vi "CSConnectGUI.panel.vi"() -> ()   [LabVIEW 2014, in "CSConnectGUI.lvlib"]
doc: "GUI for the CSConnector class (and its children)\n\nauthor: Dennis Neidherr, GSI\nlicense: GPL"
uses:
  CSConnectGUI.lvlib
  CSlibraries-extern/DimLVEvent/DimIndicators/DimIndicators.numericType.ctl
  CSlibraries-extern/DimLVEvent/DimIndicators/DimIndicators.anyType.ctl
  CSlibraries-extern/DimLVEvent/DimIndicators/DimIndicators.numericArrayType.ctl
  CSlibraries/UtilityLib/UtilityLib.valueStatus.ctl
  CSlibraries/UtilityLib/UtilityLib.helpType.ctl
  CSCore/CSSystem/CoreLib/CoreLib.short 2 byte array.vi
  CSCore/CSSystem/CoreLib/CoreLib.double 2 byte array.vi
  CSCore/CSSystem/CoreLib/CoreLib.lvlib
  CSlibraries/UtilityLib/UtilityLib.lvlib
  CSlibraries-extern/DimLVEvent/DimIndicators/DimIndicators.lvlib
  CSCore/CSApplicationBaseClasses/DeviceBase/DeviceBase.lvlib
  CSCore/GUIs/GOGUserGUIs/DeviceBaseGUI/DeviceBaseGUI.lvlib
  CSCore/CSObj/CSObj.lvlib
  CSlibraries-extern/DimLVEvent/LVDimInterface/LVDimInterface.lvlib
panel:
  in  "actStatus15":T1
  in  "actStatus14":T1
  in  "actStatus13":T1
  in  "actStatus12":T1
  in  "actStatus11":T1
  in  "actStatus10":T1
  in  "actStatus9":T1
  in  "actStatus8":T1
  in  "actStatus7":T1
  in  "actStatus6":T1
  in  "actStatus5":T1
  in  "actStatus4":T1
  in  "actStatus3":T1
  in  "actStatus2":T1
  in  "actStatus1":T1
  in  "actStatus0":T1
  out "channelIndex":u16
  in  "nomOutVoltages15":T1
  in  "nomOutVoltages14":T1
  in  "nomOutVoltages13":T1
  in  "nomOutVoltages12":T1
  in  "nomOutVoltages11":T1
  in  "nomOutVoltages10":T1
  in  "nomOutVoltages9":T1
  in  "nomOutVoltages8":T1
  in  "nomOutVoltages7":T1
  in  "nomOutVoltages6":T1
  in  "nomOutVoltages5":T1
  in  "nomOutVoltages4":T1
  in  "nomOutVoltages3":T1
  in  "nomOutVoltages2":T1
  in  "nomOutVoltages1":T1
  in  "nomOutVoltages0":T1
  in  "actOutVoltages15":T1
  in  "actOutVoltages14":T1
  in  "actOutVoltages13":T1
  in  "actOutVoltages12":T1
  in  "actOutVoltages11":T1
  in  "actOutVoltages10":T1
  in  "actOutVoltages9":T1
  in  "actOutVoltages8":T1
  in  "actOutVoltages7":T1
  in  "actOutVoltages6":T1
  in  "actOutVoltages5":T1
  in  "actOutVoltages4":T1
  in  "actOutVoltages3":T1
  in  "actOutVoltages2":T1
  in  "actOutVoltages1":T1
  in  "actOutVoltages0":T1
  in  "function":u16(ring)
  in  "EmergencyOff":bool
  in  "Set":bool
  in  "inc":dbl
  in  "setValue":dbl format="%^#_9e"
  out "ErrorString":string
  out "Busy":bool
  in  "logicalNames":T2 caption="dic_service_anyType"
  in  "nofChannels":T3 caption="dic_service_numeric"
  in  "nomVoltage":T1 caption="dic_service_numericArray"
  out "deviceIDString":string
  in  "tab":enum32{"standard"}(tab)
  in  "standardDisplay":i32[](listbox)
  in  "minus":bool
  in  "plus":bool
  out "loop counter":i32
  out "error out":errorcluster
  in  "error in (no error)":errorcluster
  in  "object ref":refnum<vi>
  in  "state":T3 caption="dic_service_numeric"
  in  "deviceID":T2 caption="dic_service_anyType"
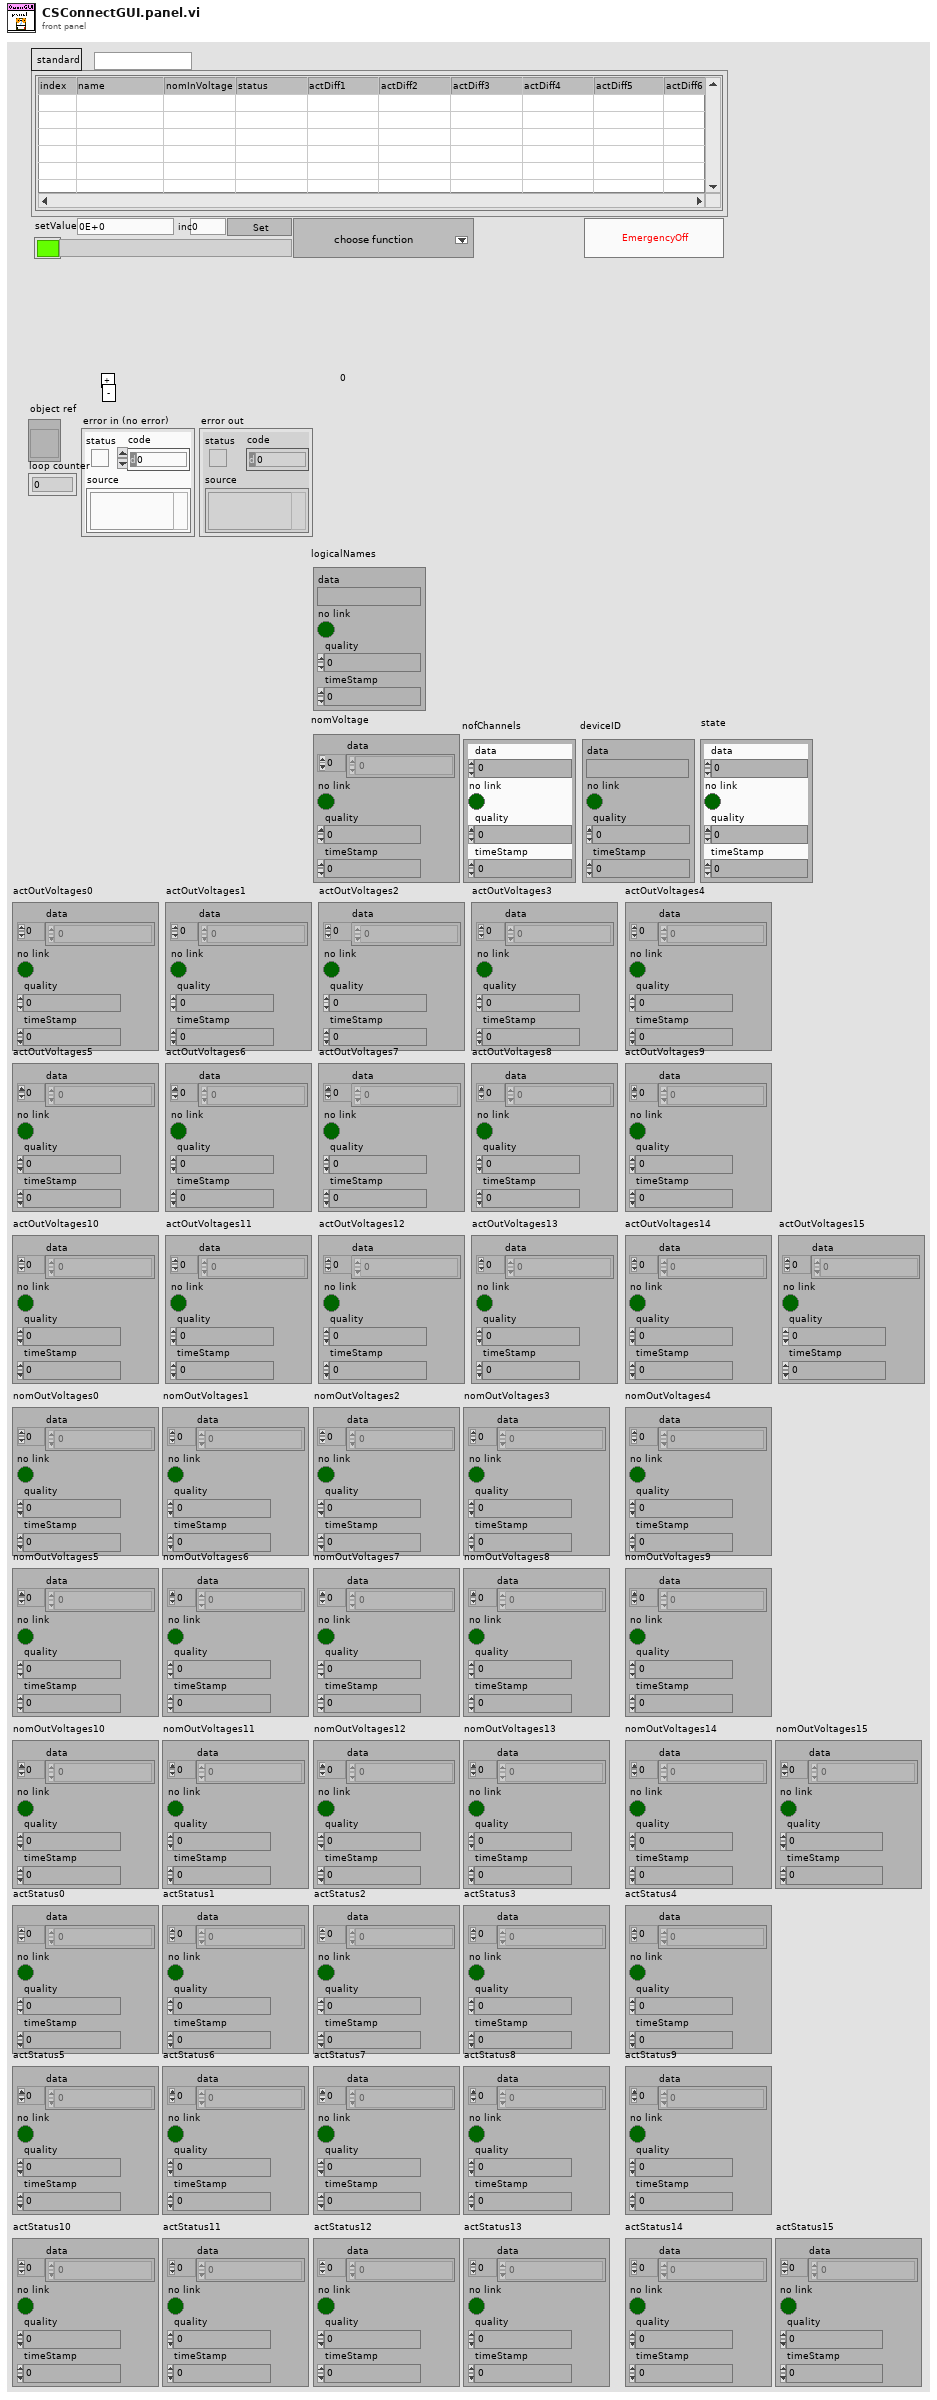
[diagram p1: front panel]
types:
  T1 = typedef "DimIndicators.lvlib/DimIndicators.numericArrayType.ctl" = cluster{"data":dbl[], "no link":bool, "quality":i32, "timeStamp":dbl}
  T2 = typedef "DimIndicators.lvlib/DimIndicators.anyType.ctl" = cluster{"data":string, "no link":bool, "quality":i32, "timeStamp":dbl}
  T3 = typedef "DimIndicators.lvlib/DimIndicators.numericType.ctl" = cluster{"data":dbl, "no link":bool, "quality":i32, "timeStamp":dbl}
  T4 = typedef "UtilityLib.lvlib/UtilityLib.valueStatus.ctl" = enum16{"no info available", "stand by/off", "on", "warning", "alarm/malfunction", "not implemented", "user action required", "important information", "system default", "control default", "indicator default", "button default"}
  T5 = cluster{"ObjectIndex":i32, "OutChannelIndex":i32}
  T6 = typedef "UtilityLib.lvlib/UtilityLib.helpType.ctl" = enum16{"unknown", "menu", "description", "about", "special0", "special1", "special2"}
  T7 = cluster{"ObjectName":string, "Indizes":cluster{"Index":i32, "Position in Matrix":i32}[]}[]
  T8 = typedef "DeviceBaseGUI.lvlib/DeviceBaseGUI.i attribute.ctl" = cluster{"GOGFrontPanel.i attribute":T9}
  T9 = typedef "GOGFrontPanel.lvlib/GOGFrontPanel.i attribute.ctl" = cluster{"GOGObject":string, "Object":string, "Method":string, "Descriptor":T10, "Input Descriptor":string, "Output Descriptor":string, "inputNames":string[], "outputNames":string[], "Values":cluster{"descriptor":string, "value":string}[]}
  T10 = typedef "BaseProcess.lvlib/BaseProcess.descriptor string definition.ctl" = string
  T11 = cluster{"ObjectName":string, "Indizes":cluster{"Index":i32, "Position in Matrix":i32}[]}
  T12 = typedef "LVRectTypeDef.ctl" = cluster{"Left":i16, "Top":i16, "Right":i16, "Bottom":i16}
  T13 = typedef "CoreDefs.rawDataType.ctl" = i8[]
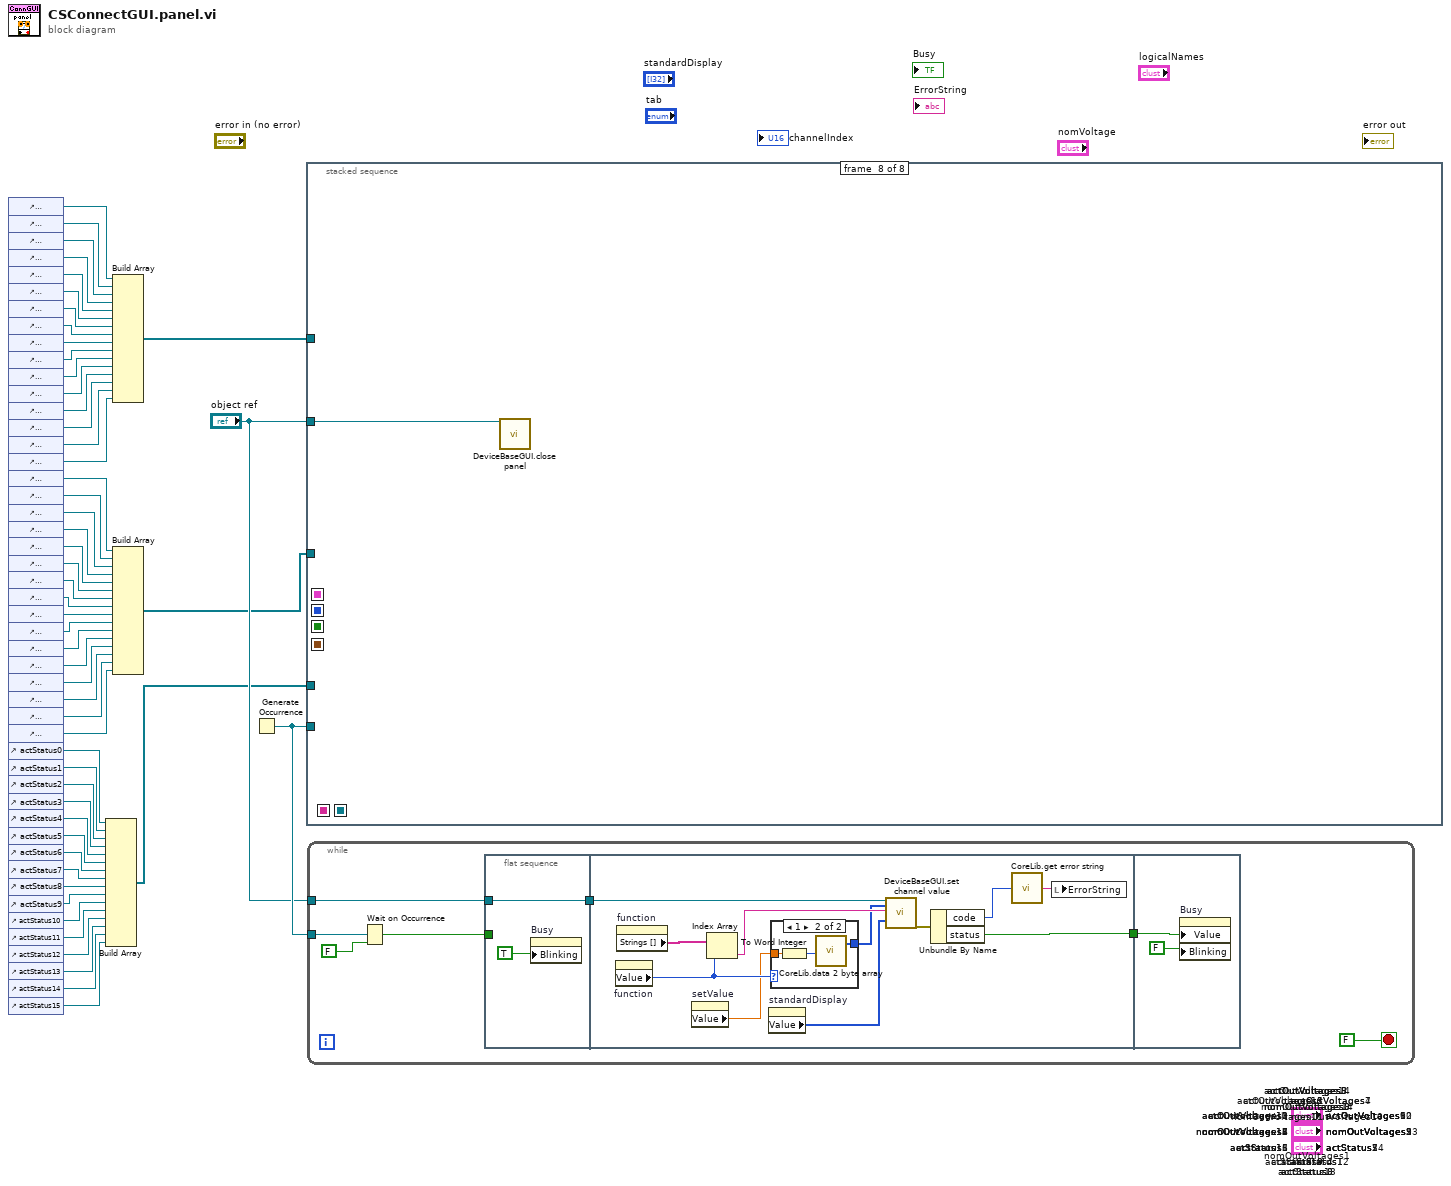
[diagram p0: block diagram]
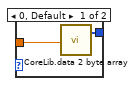
[diagram p2: hidden frame]
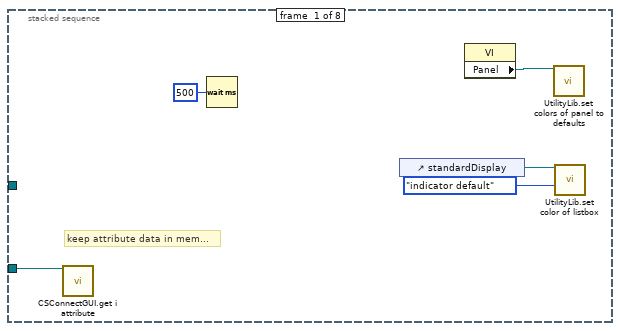
[diagram p3: hidden frame]
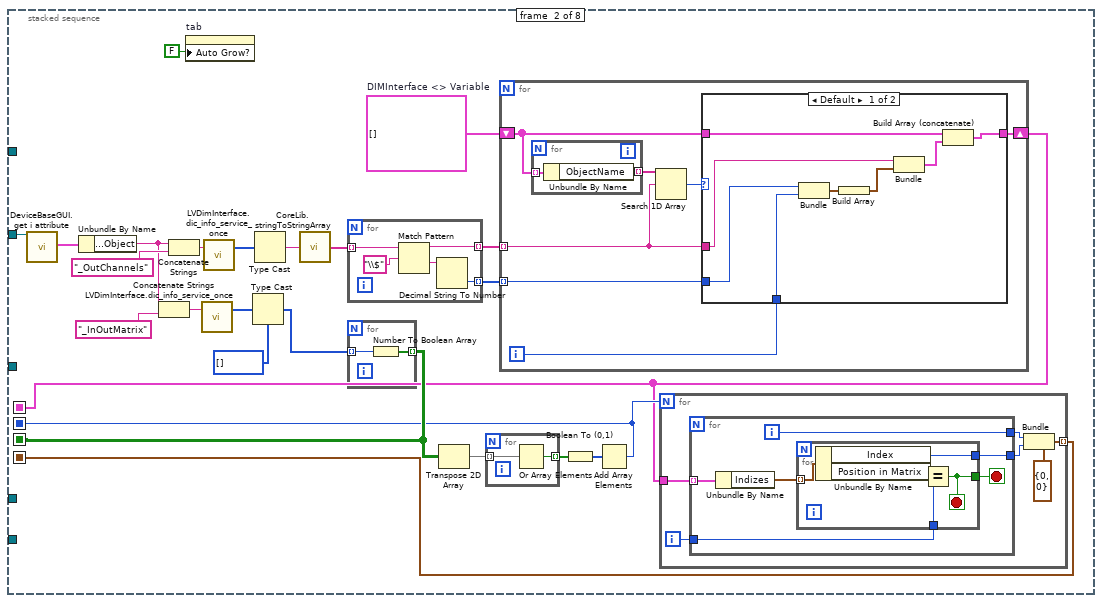
[diagram p4: hidden frame]
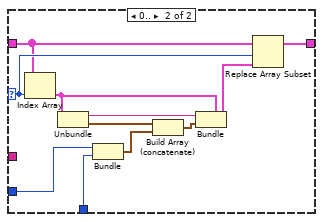
[diagram p5: hidden frame]
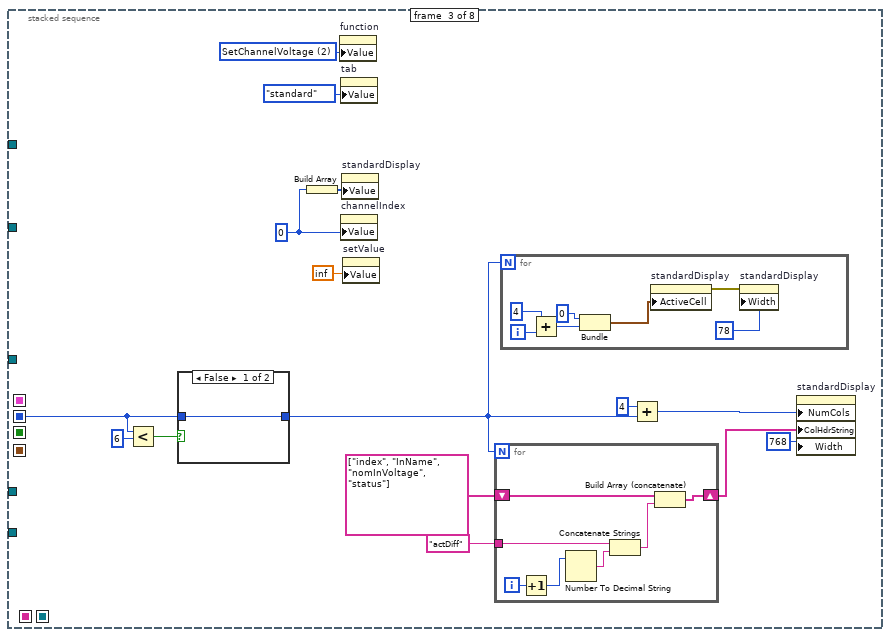
[diagram p6: hidden frame]
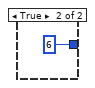
[diagram p7: hidden frame]
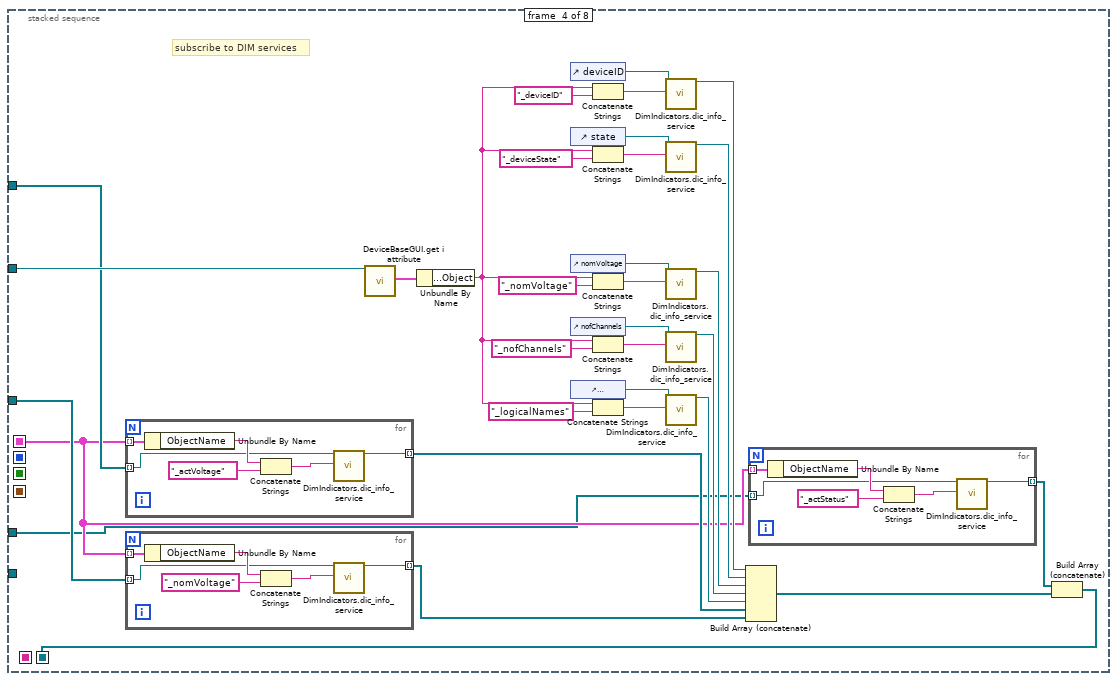
[diagram p8: hidden frame]
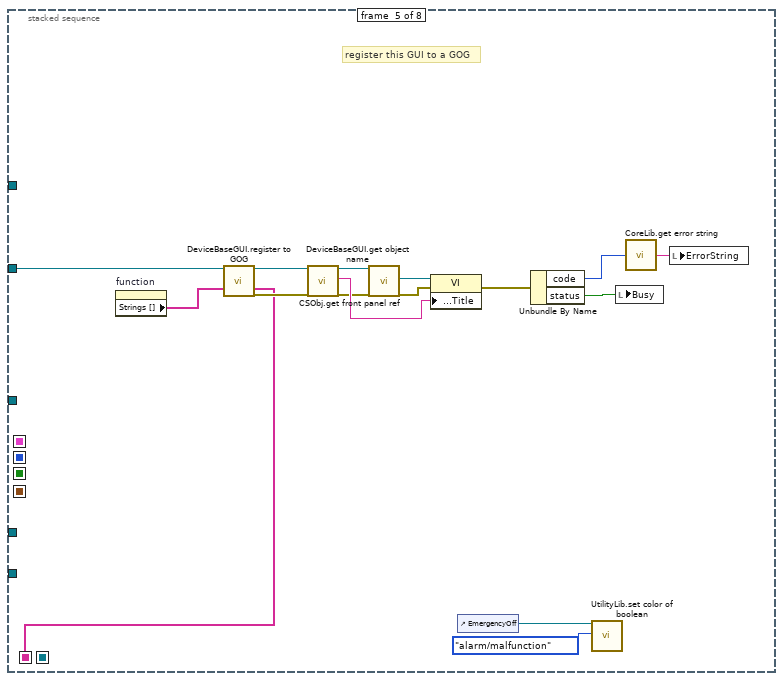
[diagram p9: hidden frame]
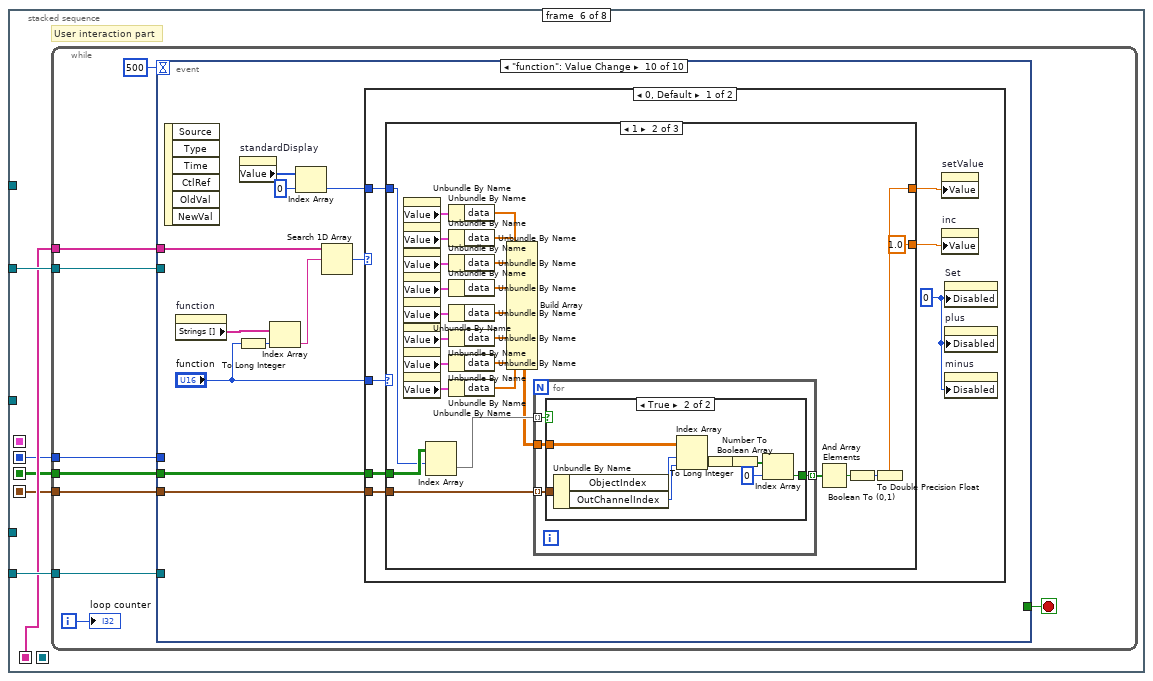
[diagram p10: hidden frame]
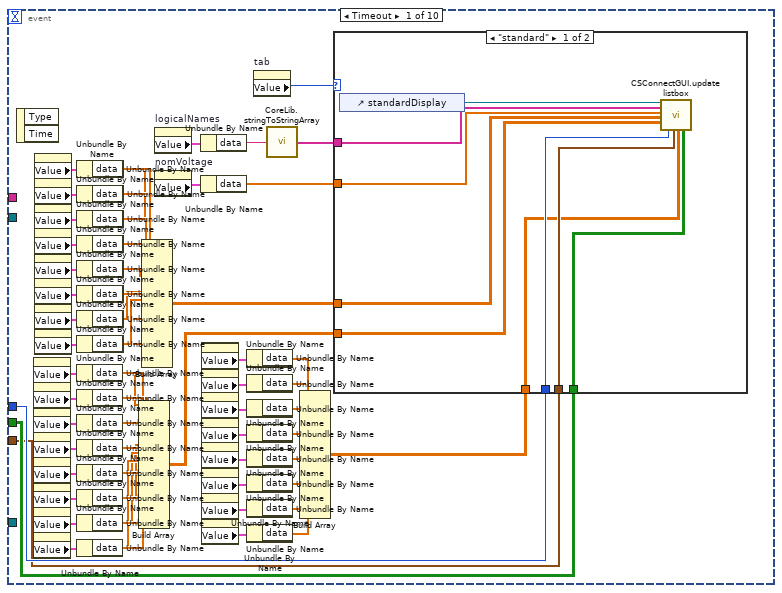
[diagram p11: hidden frame]
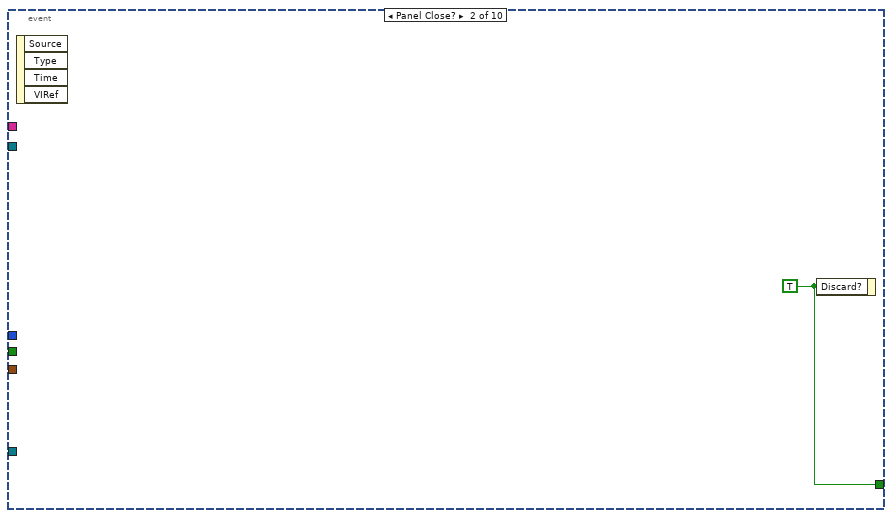
[diagram p13: hidden frame]
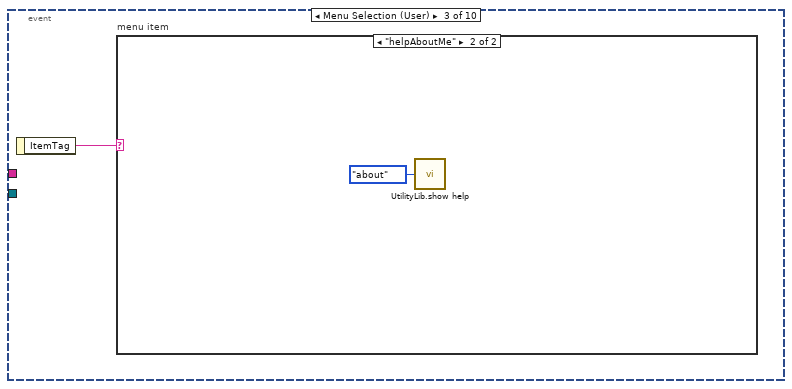
[diagram p14: hidden frame]
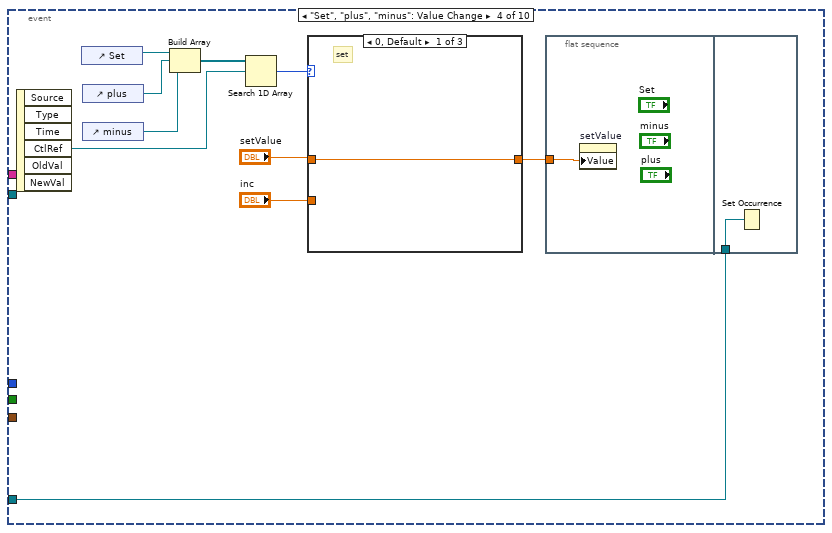
[diagram p16: hidden frame]
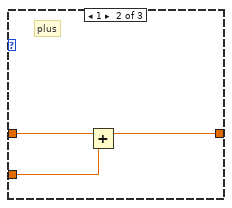
[diagram p17: hidden frame]
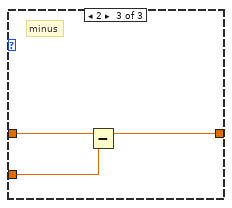
[diagram p18: hidden frame]
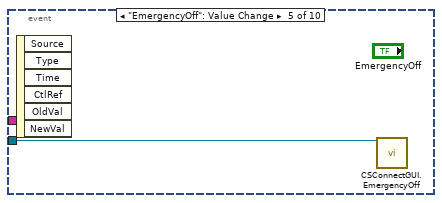
[diagram p19: hidden frame]
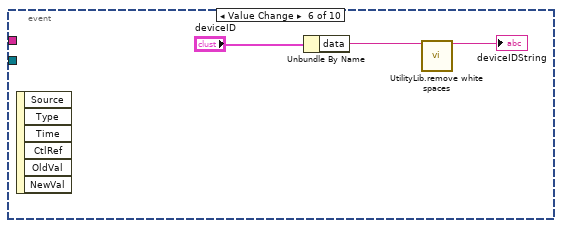
[diagram p20: hidden frame]
diagram:
  n1 = control-ref of="actOutVoltages0"() -> (w51:refnum<vi>)
  n2 = control-ref of="actOutVoltages1"() -> (w50:refnum<vi>)
  n3 = control-ref of="actOutVoltages2"() -> (w49:refnum<vi>)
  n4 = control-ref of="actOutVoltages3"() -> (w48:refnum<vi>)
  n5 = control-ref of="actOutVoltages4"() -> (w47:refnum<vi>)
  n6 = control-ref of="actOutVoltages5"() -> (w46:refnum<vi>)
  n7 = control-ref of="actOutVoltages6"() -> (w45:refnum<vi>)
  n8 = control-ref of="actOutVoltages7"() -> (w44:refnum<vi>)
  n9 = control-ref of="actOutVoltages8"() -> (w43:refnum<vi>)
  n10 = control-ref of="actOutVoltages9"() -> (w42:refnum<vi>)
  n11 = control-ref of="actOutVoltages10"() -> (w41:refnum<vi>)
  n12 = control-ref of="actOutVoltages11"() -> (w36:refnum<vi>)
  n13 = control-ref of="actOutVoltages12"() -> (w37:refnum<vi>)
  n14 = control-ref of="actOutVoltages13"() -> (w38:refnum<vi>)
  n15 = control-ref of="actOutVoltages14"() -> (w39:refnum<vi>)
  n16 = control-ref of="actOutVoltages15"() -> (w40:refnum<vi>)
  n17 = control-ref of="nomOutVoltages0"() -> (w34:refnum<vi>)
  n18 = control-ref of="nomOutVoltages1"() -> (w33:refnum<vi>)
  n19 = control-ref of="nomOutVoltages2"() -> (w32:refnum<vi>)
  n20 = control-ref of="nomOutVoltages3"() -> (w31:refnum<vi>)
  n21 = control-ref of="nomOutVoltages4"() -> (w30:refnum<vi>)
  n22 = control-ref of="nomOutVoltages5"() -> (w29:refnum<vi>)
  n23 = control-ref of="nomOutVoltages6"() -> (w28:refnum<vi>)
  n24 = control-ref of="nomOutVoltages7"() -> (w27:refnum<vi>)
  n25 = control-ref of="nomOutVoltages8"() -> (w26:refnum<vi>)
  n26 = control-ref of="nomOutVoltages9"() -> (w19:refnum<vi>)
  n27 = control-ref of="nomOutVoltages10"() -> (w20:refnum<vi>)
  n28 = control-ref of="nomOutVoltages11"() -> (w21:refnum<vi>)
  n29 = control-ref of="nomOutVoltages12"() -> (w22:refnum<vi>)
  n30 = control-ref of="nomOutVoltages13"() -> (w23:refnum<vi>)
  n31 = control-ref of="nomOutVoltages14"() -> (w24:refnum<vi>)
  n32 = control-ref of="nomOutVoltages15"() -> (w25:refnum<vi>)
  n33 = control-ref of="actStatus0"() -> (w17:refnum<vi>)
  n34 = control-ref of="actStatus1"() -> (w16:refnum<vi>)
  n35 = control-ref of="actStatus2"() -> (w15:refnum<vi>)
  n36 = control-ref of="actStatus3"() -> (w14:refnum<vi>)
  n37 = control-ref of="actStatus4"() -> (w13:refnum<vi>)
  n38 = control-ref of="actStatus5"() -> (w12:refnum<vi>)
  n39 = control-ref of="actStatus6"() -> (w11:refnum<vi>)
  n40 = control-ref of="actStatus7"() -> (w10:refnum<vi>)
  n41 = control-ref of="actStatus8"() -> (w9:refnum<vi>)
  n42 = control-ref of="actStatus9"() -> (w2:refnum<vi>)
  n43 = control-ref of="actStatus10"() -> (w3:refnum<vi>)
  n44 = control-ref of="actStatus11"() -> (w4:refnum<vi>)
  n45 = control-ref of="actStatus12"() -> (w5:refnum<vi>)
  n46 = control-ref of="actStatus13"() -> (w6:refnum<vi>)
  n47 = control-ref of="actStatus14"() -> (w7:refnum<vi>)
  n48 = control-ref of="actStatus15"() -> (w8:refnum<vi>)
  n49 = Build Array(w17, w16, w15, w14, w13, w12, w11, w10, w9, w2, w3, w4, w5, w6, w7, w8) -> (w1:refnum<vi>[])
  n50 = Build Array(w51, w50, w49, w48, w47, w46, w45, w44, w43, w42, w41, w36, w37, w38, w39, w40) -> (w35:refnum<vi>[])
  n51 = Build Array(w34, w33, w32, w31, w30, w29, w28, w27, w26, w19, w20, w21, w22, w23, w24, w25) -> (w18:refnum<vi>[])
  n52 = Generate Occurrence() -> (w53:refnum<k4>)
  n53 = stacked-sequence {
    seq-local: [_ _ _ w198 _ _ _ _] -> [_ _ _ _ _ _ w526 _]
    seq-local: [_ _ _ _ w218 _ _ _] -> [_ _ _ _ _ w237 _ _]
    seq-local: [_ w61 _ _ _ _ _ _] -> [_ _ _ w169 _ _ _ _]
    seq-local: [_ w62 _ _ _ _ _ _] -> [_ _ w139 _ _ w236 _ _]
    seq-local: [_ w63 _ _ _ _ _ _] -> [_ _ _ _ _ w235 _ _]
    seq-local: [_ w60 _ _ _ _ _ _] -> [_ _ _ _ _ w234 _ _]
    tunnel: "object ref" -> [w54 w81 _ w199 w224 w239 _ w528]
    tunnel: w53 -> [_ _ _ _ _ w238 _ _]
    tunnel: w35 -> [_ _ _ w176 _ _ _ _]
    tunnel: w18 -> [_ _ _ w172 _ _ _ _]
    tunnel: w1 -> [_ _ _ w168 _ _ _ _]
    frame #0 {
      # "keep attribute data in mem..."
      n54 = call "CSConnectGUI.get i attribute.vi"("i ref in"=w54) -> ()  [unwired: 16 in, 3 out]
      n55 = Wait (ms)(milliseconds to wait=u32 500) -> ()  [unwired: 1 out]
      n56 = control-ref of="standardDisplay"() -> (w56:refnum<vi>)
      n57 = property on="Property Node" class="VI"() -> ("Panel"=w55:refnum<vi>)  [unwired: 2 in, 2 out]
      n58 = call "UtilityLib.set colors of panel to defaults.vi"("Front Panel"=w55) -> ()  [unwired: 18 in, 1 out]
      n59 = call "UtilityLib.set color of listbox.vi"("listboxRef"=w56, "valueStatus"=UtilityLib.valueStatus."indicator default") -> ()  [unwired: 17 in, 1 out]
    }
    frame #1 {
      w74 = T7 []  # DIMInterface <> Variable
      n60 = call "DeviceBaseGUI.get i attribute.vi"("i ref in"=w81) -> ("i attribute"=w82:T8)  [unwired: 16 in, 2 out]
      n61 = Unbundle By Name(w82) -> ("GOGFrontPanel.i attribute.Object"=w71:string)
      n62 = Concatenate Strings(w71, "_InOutMatrix" ("string")) -> (w73:string)
      n63 = Concatenate Strings(w71, "_OutChannels" ("string")) -> (w80:string)
      n64 = property on="tab" class="TabCtl (strict)"("Auto Grow?"=FALSE) -> ()  [unwired: 2 in, 2 out]
      n65 = call "LVDimInterface.dic_info_service_once.vi"("serviceName"=w73) -> ("data"=w70:i8[])  [unwired: 15 in, 3 out]
      n66 = call "LVDimInterface.dic_info_service_once.vi"("serviceName"=w80) -> ("data"=w78:i8[])  [unwired: 15 in, 3 out]
      n67 = Type Cast(type=i32[] [] ("32bit integer"), x=w70) -> (*(type *) &x=w68:i32[])
      n68 = Type Cast(x=w78) -> (*(type *) &x=w77:string)  [unwired: 1 in]
      n69 = call "CoreLib.stringToStringArray.vi"("String"=w77) -> ("Array"=w76:string[])
      n70 = for {
        tunnel: w76 -> [w136] mode=indexing
        tunnel: [w132] -> w67 mode=indexing
        tunnel: [w133] -> w75 mode=indexing
        n71 = Match Pattern(string=w136, regular expression="\\$") -> (before substring=w132:string, after substring=w134:string)  [unwired: 1 in, 2 out]
        n72 = Decimal String To Number(string=w134) -> (number=w133:i32)  [unwired: 2 in, 1 out]
      }
      n73 = for {
        tunnel: w68 -> [w103] mode=indexing
        tunnel: [w102] -> w63 mode=indexing
        n74 = Number To Boolean Array(number=w103) -> (Boolean array=w102:bool[])
      }
      n75 = Transpose 2D Array(2D array=w63) -> (transposed array=w66:bool[][])
      n76 = for {
        tunnel: w66 -> [w101] mode=indexing
        tunnel: [w100] -> w64 mode=indexing
        n77 = Or Array Elements(Boolean array=w101) -> (logical OR=w100:bool)
      }
      n78 = for {
        tunnel: w67 -> [w106] mode=indexing
        tunnel: w75 -> [w105] mode=indexing
        shift-right: [w107] -> w61
        shift-left: w74 -> [w108]
        i -> [w104]
        n79 = for {
          tunnel: w108 -> [w131] mode=indexing
          tunnel: [w130] -> w110 mode=indexing
          n80 = Unbundle By Name(w131) -> ("ObjectName"=w130:string)
        }
        n81 = Search 1D Array(1D array=w110, element=w106) -> (index of element=w109:i32)  [unwired: 1 in]
        n82 = case shown="Default" w109 {
          selector: w109 -> [_ w128]
          tunnel: w108 -> [w118 w127]
          tunnel: [w117 w129] -> w107
          tunnel: w106 -> [w115 _]
          tunnel: w105 -> [w112 w120]
          tunnel: w104 -> [w111 w119]
          frame Default {
            n83 = Bundle(w112, w111) -> (w114:cluster{i32, i32})  [unwired: 1 in]
            n84 = Build Array(w114) -> (w113:cluster{i32, i32}[])
            n85 = Bundle(w115, w113) -> (w116:cluster{string, cluster{i32, i32}[]})  [unwired: 1 in]
            n86 = Build Array (concatenate)(w118, w116) -> (w117:T7)
          }
          frame 0.. {
            n87 = Index Array(array=w127, index=w128) -> (element=w126:T11)
            n88 = Unbundle(w126) -> ("ObjectName"=w125:string, "Indizes"=w122:cluster{"Index":i32, "Position in Matrix":i32}[])
            n89 = Bundle(w120, w119) -> (w121:cluster{i32, i32})  [unwired: 1 in]
            n90 = Build Array (concatenate)(w122, w121) -> (w124:cluster{"Index":i32, "Position in Matrix":i32}[])
            n91 = Bundle(cluster=w126, "ObjectName"=w125, "Indizes"=w124) -> (w123:T11)
            n92 = Replace Array Subset(array=w127, new element=w123, index=w128) -> (w129:T7)
          }
        }
      }
      n93 = Boolean To (0,1)(Boolean=w64) -> (0, 1=w65:i16[])
      n94 = Add Array Elements(numeric array=w65) -> (sum=w62:i16)
      n95 = for {
        N: w62 -> [_]
        tunnel: w61 -> [w88]
        tunnel: [w84] -> w60 mode=indexing
        i -> [w87]
        n96 = for {
          tunnel: w88 -> [w94] mode=indexing
          tunnel: [w89] -> w86
          tunnel: [w92] -> w85
          tunnel: w87 -> [w90]
          i -> [w89]
          stop <- w91 stop-if-true
          n97 = Unbundle By Name(w94) -> ("Indizes"=w93:cluster{"Index":i32, "Position in Matrix":i32}[])
          n98 = for {
            tunnel: w93 -> [w99] mode=indexing
            tunnel: [w97] -> w91
            tunnel: [w96] -> w92
            tunnel: w90 -> [w95]
            stop <- w97 stop-if-true
            n99 = Unbundle By Name(w99) -> ("Index"=w96:i32, "Position in Matrix"=w98:i32)
            n100 = Equal?(x=w98, y=w95) -> (x = y?=w97:bool)
          }
        }
        n101 = Bundle(cluster=T5 {"ObjectIndex"=0, "OutChannelIndex"=0}, "ObjectIndex"=w86, "OutChannelIndex"=w85) -> (w84:T5)
      }
    }
    frame #2 {
      w148 = 0
      w151 = u16 2 items=["choose function", "SetChannelOnOff", "SetChannelVoltage", "SetChannelCurrent", "SetChannelTripCurrent", "SetChannelRampUpSpeed", "SetChannelRampDownSpeed", "GetChannelOnOff", "GetChannelVoltage", "GetChannelCurrent", "GetChannelTripCurrent", "GetChannelRampUpSpeed", "GetChannelRampDownSpeed", "GetChannelStatus", "Reset"] ("function")
      n102 = Less?(x=w139, y=6) -> (x < y?=w140:bool)
      n103 = case shown="False" w140 {
        tunnel: w139 -> [w159 _]
        tunnel: [w159 6] -> w137
        frame False {
        }
        frame True {
        }
      }
      n104 = Build Array(w148) -> (w150:i32[])
      n105 = property on="function" class="Ring (strict)"("Value"=w151) -> ()  [unwired: 2 in, 2 out]
      n106 = property on="tab" class="TabCtl (strict)"("Value"=enum32{"standard"}."standard" ("tab")) -> ()  [unwired: 2 in, 2 out]
      n107 = property on="channelIndex" class="DigNum (strict)"("Value"=w148) -> ()  [unwired: 2 in, 2 out]
      n108 = property on="standardDisplay" class="MCListbox (strict)"("Value"=w150) -> ()  [unwired: 2 in, 2 out]
      n109 = property on="setValue" class="DigNum (strict)"("Value"=inf ("Positive Infinity")) -> ()  [unwired: 2 in, 2 out]
      n110 = for {
        N: w137 -> [_]
        shift-right: [w166] -> w142
        shift-left: string[] ["index", "InName", "nomInVoltage", "status"] -> [w167]
        tunnel: "actDiff" -> [w165]
        i -> [w162]
        n111 = Increment(x=w162) -> (x+1=w161:i32)
        n112 = Number To Decimal String(number=w161) -> (decimal integer string=w163:string)  [unwired: 1 in]
        n113 = Concatenate Strings(w165, w163) -> (w164:string)
        n114 = Build Array (concatenate)(w167, w164) -> (w166:string[])
      }
      n115 = for {
        N: w137 -> [_]
        i -> [w156]
        n116 = Add(x=4, y=w156) -> (x+y=w154:i32)
        n117 = Bundle(0, w154) -> (w152:cluster{i32, i32})  [unwired: 1 in]
        n118 = property on="standardDisplay" class="MCListbox (strict)"("ActiveCell"=w152) -> (error out=w158:errorcluster)  [unwired: 2 in, 1 out]
        n119 = property on="standardDisplay" class="MCListbox (strict)"(error in=w158, "Width"=u32 78 ("Active Cell:Cell Size:Width")) -> ()  [unwired: 1 in, 2 out]
      }
      n120 = Add(x=i16 4, y=w137) -> (x+y=w146:i32)
      n121 = property on="standardDisplay" class="MCListbox (strict)"("NumCols"=w146, "ColHdrString"=w142, "Width"=u32 768 ("Size:Width")) -> ()  [unwired: 2 in, 2 out]
    }
    frame #3 {
      # "subscribe to DIM services"
      n122 = for {
        tunnel: w169 -> [w215] mode=indexing
        tunnel: w176 -> [w213] mode=indexing
        tunnel: [w212] -> w175 mode=indexing
        n123 = Unbundle By Name(w215) -> ("ObjectName"=w214:string)
        n124 = Concatenate Strings(w214, "_actVoltage" ("string")) -> (w216:string)
        n125 = call "DimIndicators.dic_info_service.vi"("controlRef"=w213, "serviceName"=w216) -> ("controlRef out"=w212:refnum<vi>)  [unwired: 16 in, 1 out]
      }
      n126 = for {
        tunnel: w169 -> [w209] mode=indexing
        tunnel: w172 -> [w207] mode=indexing
        tunnel: [w206] -> w171 mode=indexing
        n127 = Unbundle By Name(w209) -> ("ObjectName"=w208:string)
        n128 = Concatenate Strings(w208, "_nomVoltage" ("string")) -> (w210:string)
        n129 = call "DimIndicators.dic_info_service.vi"("controlRef"=w207, "serviceName"=w210) -> ("controlRef out"=w206:refnum<vi>)  [unwired: 16 in, 1 out]
      }
      n130 = call "DeviceBaseGUI.get i attribute.vi"("i ref in"=w199) -> ("i attribute"=w196:T8)  [unwired: 16 in, 2 out]
      n131 = Unbundle By Name(w196) -> ("GOGFrontPanel.i attribute.Object"=w191:string)
      n132 = control-ref of="deviceID"() -> (w189:refnum<vi>)
      n133 = control-ref of="state"() -> (w187:refnum<vi>)
      n134 = control-ref of="nomVoltage"() -> (w185:refnum<vi>)
      n135 = control-ref of="nofChannels"() -> (w183:refnum<vi>)
      n136 = control-ref of="logicalNames"() -> (w181:refnum<vi>)
      n137 = Concatenate Strings(w191, "_deviceID" ("string")) -> (w190:string)
      n138 = Concatenate Strings(w191, "_deviceState" ("string")) -> (w188:string)
      n139 = Concatenate Strings(w191, "_nomVoltage" ("string")) -> (w186:string)
      n140 = Concatenate Strings(w191, "_nofChannels" ("string")) -> (w184:string)
      n141 = Concatenate Strings(w191, "_logicalNames" ("string")) -> (w182:string)
      n142 = call "DimIndicators.dic_info_service.vi"("controlRef"=w189, "serviceName"=w190) -> ("controlRef out"=w173:refnum<vi>)  [unwired: 16 in, 1 out]
      n143 = call "DimIndicators.dic_info_service.vi"("controlRef"=w187, "serviceName"=w188) -> ("controlRef out"=w174:refnum<vi>)  [unwired: 16 in, 1 out]
      n144 = call "DimIndicators.dic_info_service.vi"("controlRef"=w185, "serviceName"=w186) -> ("controlRef out"=w180:refnum<vi>)  [unwired: 16 in, 1 out]
      n145 = call "DimIndicators.dic_info_service.vi"("controlRef"=w183, "serviceName"=w184) -> ("controlRef out"=w179:refnum<vi>)  [unwired: 16 in, 1 out]
      n146 = call "DimIndicators.dic_info_service.vi"("controlRef"=w181, "serviceName"=w182) -> ("controlRef out"=w178:refnum<vi>)  [unwired: 16 in, 1 out]
      n147 = Build Array (concatenate)(w173, w174, w180, w179, w178, w175, w171) -> (w177:refnum<vi>[])
      n148 = for {
        tunnel: w169 -> [w203] mode=indexing
        tunnel: w168 -> [w201] mode=indexing
        tunnel: [w200] -> w170 mode=indexing
        n149 = Unbundle By Name(w203) -> ("ObjectName"=w202:string)
        n150 = Concatenate Strings(w202, "_actStatus" ("string")) -> (w204:string)
        n151 = call "DimIndicators.dic_info_service.vi"("controlRef"=w201, "serviceName"=w204) -> ("controlRef out"=w200:refnum<vi>)  [unwired: 16 in, 1 out]
      }
      n152 = Build Array (concatenate)(w170, w177) -> (w198:refnum<vi>[])
    }
    frame #4 {
      # "register this GUI to a GOG"
      n153 = property on="function" class="Ring (strict)"() -> ("Strings []"=w223:string[])  [unwired: 2 in, 2 out]
      n154 = call "DeviceBaseGUI.register to GOG.vi"("i ref in"=w224, "myMethods"=w223) -> ("i ref out"=w227:refnum<vi>, "configuredMethods"=w218:string[], "error out"=w226:errorcluster)  [unwired: 15 in]
      n155 = call "DeviceBaseGUI.get object name.vi"("i ref in"=w227, "error in (no error)"=w226) -> ("i ref out"=w228:refnum<vi>, "objectName"=w231:string, "error out"=w229:errorcluster)  [unwired: 15 in]
      n156 = call "CSObj.get front panel ref.vi"("i ref in"=w228, "error in (no error)"=w229) -> ("frontPanelRef"=w225:refnum<vi>, "error out"=w230:errorcluster)  [unwired: 15 in, 1 out]
      n157 = property class="VI"(reference=w225, error in=w230, "Front Panel Window:Title"=w231) -> (error out=w222:errorcluster)  [unwired: 1 out]
      n158 = control-ref of="EmergencyOff"() -> (w233:refnum<vi>)
      n159 = Unbundle By Name(w222) -> ("code"=w221:i32, "status"=w219:bool)
      n160 = call "UtilityLib.set color of boolean.vi"("button"=w233, "valueStatus"=UtilityLib.valueStatus."alarm/malfunction") -> ()  [unwired: 17 in, 1 out]
      n161 = local write "Busy"(w219) -> ()
      n162 = call "CoreLib.get error string.vi"("Error Code"=w221) -> ("Error String"=w220:string)
      n163 = local write "ErrorString"(w220) -> ()
    }
    frame #5 {
      # "User interaction part"
      n164 = while {
        tunnel: w239 -> [w246]
        tunnel: w238 -> [w244]
        tunnel: w237 -> [w243]
        tunnel: w236 -> [w242]
        tunnel: w235 -> [w241]
        tunnel: w234 -> [w240]
        i -> [w247]
        stop <- w248 stop-if-true
        n165 = event shown="[9] \"function\": Value Change" {
          selector: _ -> [_ _ _ _ _ _ _ _ _ _]
          dyn-events: _ -> [_ _ _ _ _ _ _ _ _ _]
          timeout: 500 -> [_ _ _ _ _ _ _ _ _ _]
          tunnel: [_ w366 _ _ _ _ _ _ _ _] -> w248
          tunnel: w246 -> [_ _ _ _ w388 _ _ _ _ _]
          tunnel: w244 -> [_ _ _ w369 _ _ _ _ _ _]
          tunnel: w243 -> [_ _ _ _ _ _ _ _ _ w443]
          tunnel: w242 -> [w317 _ _ _ _ _ _ _ _ _]
          tunnel: w241 -> [w316 _ _ _ _ _ _ _ _ w441]
          tunnel: w240 -> [w315 _ _ _ _ _ _ _ _ w440]
          event Timeout {
            n166 = event-data() -> ()  [unwired: 1 in, 2 out]
            n167 = property on="nomOutVoltages0" class="Clust (strict)"() -> ("Value"=w283:T1)  [unwired: 2 in, 2 out]
            n168 = property on="nomOutVoltages8" class="Clust (strict)"() -> ("Value"=w291:T1)  [unwired: 2 in, 2 out]
            n169 = property on="nomOutVoltages1" class="Clust (strict)"() -> ("Value"=w284:T1)  [unwired: 2 in, 2 out]
            n170 = property on="nomOutVoltages9" class="Clust (strict)"() -> ("Value"=w292:T1)  [unwired: 2 in, 2 out]
            n171 = property on="nomOutVoltages2" class="Clust (strict)"() -> ("Value"=w285:T1)  [unwired: 2 in, 2 out]
            n172 = property on="nomOutVoltages10" class="Clust (strict)"() -> ("Value"=w293:T1)  [unwired: 2 in, 2 out]
            n173 = property on="nomOutVoltages3" class="Clust (strict)"() -> ("Value"=w286:T1)  [unwired: 2 in, 2 out]
            n174 = property on="nomOutVoltages11" class="Clust (strict)"() -> ("Value"=w294:T1)  [unwired: 2 in, 2 out]
            n175 = property on="nomOutVoltages4" class="Clust (strict)"() -> ("Value"=w287:T1)  [unwired: 2 in, 2 out]
            n176 = property on="nomOutVoltages12" class="Clust (strict)"() -> ("Value"=w295:T1)  [unwired: 2 in, 2 out]
            n177 = property on="nomOutVoltages5" class="Clust (strict)"() -> ("Value"=w288:T1)  [unwired: 2 in, 2 out]
            n178 = property on="nomOutVoltages13" class="Clust (strict)"() -> ("Value"=w296:T1)  [unwired: 2 in, 2 out]
            n179 = property on="nomOutVoltages6" class="Clust (strict)"() -> ("Value"=w289:T1)  [unwired: 2 in, 2 out]
            n180 = property on="nomOutVoltages14" class="Clust (strict)"() -> ("Value"=w297:T1)  [unwired: 2 in, 2 out]
            n181 = property on="nomOutVoltages7" class="Clust (strict)"() -> ("Value"=w290:T1)  [unwired: 2 in, 2 out]
            n182 = property on="nomOutVoltages15" class="Clust (strict)"() -> ("Value"=w298:T1)  [unwired: 2 in, 2 out]
            n183 = property on="actOutVoltages8" class="Clust (strict)"() -> ("Value"=w335:T1)  [unwired: 2 in, 2 out]
            n184 = property on="actOutVoltages0" class="Clust (strict)"() -> ("Value"=w343:T1)  [unwired: 2 in, 2 out]
            n185 = property on="actOutVoltages9" class="Clust (strict)"() -> ("Value"=w336:T1)  [unwired: 2 in, 2 out]
            n186 = property on="actOutVoltages1" class="Clust (strict)"() -> ("Value"=w344:T1)  [unwired: 2 in, 2 out]
            n187 = property on="actOutVoltages10" class="Clust (strict)"() -> ("Value"=w337:T1)  [unwired: 2 in, 2 out]
            n188 = property on="actOutVoltages2" class="Clust (strict)"() -> ("Value"=w345:T1)  [unwired: 2 in, 2 out]
            n189 = property on="actOutVoltages11" class="Clust (strict)"() -> ("Value"=w338:T1)  [unwired: 2 in, 2 out]
            n190 = property on="actOutVoltages3" class="Clust (strict)"() -> ("Value"=w346:T1)  [unwired: 2 in, 2 out]
            n191 = property on="actOutVoltages12" class="Clust (strict)"() -> ("Value"=w339:T1)  [unwired: 2 in, 2 out]
            n192 = property on="actOutVoltages4" class="Clust (strict)"() -> ("Value"=w347:T1)  [unwired: 2 in, 2 out]
            n193 = property on="actOutVoltages13" class="Clust (strict)"() -> ("Value"=w340:T1)  [unwired: 2 in, 2 out]
            n194 = property on="actOutVoltages5" class="Clust (strict)"() -> ("Value"=w348:T1)  [unwired: 2 in, 2 out]
            n195 = property on="actOutVoltages14" class="Clust (strict)"() -> ("Value"=w341:T1)  [unwired: 2 in, 2 out]
            n196 = property on="actOutVoltages6" class="Clust (strict)"() -> ("Value"=w349:T1)  [unwired: 2 in, 2 out]
            n197 = property on="actOutVoltages15" class="Clust (strict)"() -> ("Value"=w342:T1)  [unwired: 2 in, 2 out]
            n198 = property on="actOutVoltages7" class="Clust (strict)"() -> ("Value"=w350:T1)  [unwired: 2 in, 2 out]
            n199 = Unbundle By Name(w343) -> ("data"=w334:dbl[])
            n200 = Unbundle By Name(w344) -> ("data"=w333:dbl[])
            n201 = Unbundle By Name(w345) -> ("data"=w332:dbl[])
            n202 = Unbundle By Name(w346) -> ("data"=w331:dbl[])
            n203 = Unbundle By Name(w347) -> ("data"=w330:dbl[])
            n204 = Unbundle By Name(w348) -> ("data"=w329:dbl[])
            n205 = Unbundle By Name(w349) -> ("data"=w328:dbl[])
            n206 = Unbundle By Name(w350) -> ("data"=w327:dbl[])
            n207 = Unbundle By Name(w291) -> ("data"=w307:dbl[])
            n208 = Unbundle By Name(w283) -> ("data"=w299:dbl[])
            n209 = Unbundle By Name(w292) -> ("data"=w314:dbl[])
            n210 = Unbundle By Name(w284) -> ("data"=w300:dbl[])
            n211 = Unbundle By Name(w293) -> ("data"=w313:dbl[])
            n212 = Unbundle By Name(w285) -> ("data"=w301:dbl[])
            n213 = Unbundle By Name(w294) -> ("data"=w312:dbl[])
            n214 = Unbundle By Name(w286) -> ("data"=w302:dbl[])
            n215 = Unbundle By Name(w295) -> ("data"=w311:dbl[])
            n216 = Unbundle By Name(w287) -> ("data"=w303:dbl[])
            n217 = Unbundle By Name(w296) -> ("data"=w310:dbl[])
            n218 = Unbundle By Name(w288) -> ("data"=w304:dbl[])
            n219 = Unbundle By Name(w297) -> ("data"=w309:dbl[])
            n220 = Unbundle By Name(w289) -> ("data"=w305:dbl[])
            n221 = Unbundle By Name(w298) -> ("data"=w308:dbl[])
            n222 = Unbundle By Name(w290) -> ("data"=w306:dbl[])
            n223 = Unbundle By Name(w335) -> ("data"=w326:dbl[])
            n224 = Unbundle By Name(w336) -> ("data"=w325:dbl[])
            n225 = Unbundle By Name(w337) -> ("data"=w324:dbl[])
            n226 = Unbundle By Name(w338) -> ("data"=w323:dbl[])
            n227 = Unbundle By Name(w339) -> ("data"=w322:dbl[])
            n228 = Unbundle By Name(w340) -> ("data"=w321:dbl[])
            n229 = Unbundle By Name(w341) -> ("data"=w320:dbl[])
            n230 = Unbundle By Name(w342) -> ("data"=w319:dbl[])
            n231 = Build Array(w299, w300, w301, w302, w303, w304, w305, w306, w307, w314, w313, w312, w311, w310, w309, w308) -> (w282:dbl[][])
            n232 = Build Array(w334, w333, w332, w331, w330, w329, w328, w327, w326, w325, w324, w323, w322, w321, w320, w319) -> (w318:dbl[][])
            n233 = property on="logicalNames" class="Clust (strict)"() -> ("Value"=w356:T2)  [unwired: 2 in, 2 out]
            n234 = property on="nomVoltage" class="Clust (strict)"() -> ("Value"=w353:T1)  [unwired: 2 in, 2 out]
            n235 = Unbundle By Name(w356) -> ("data"=w355:string)
            n236 = Unbundle By Name(w353) -> ("data"=w352:dbl[])
            n237 = property on="actStatus0" class="Clust (strict)"() -> ("Value"=w250:T1)  [unwired: 2 in, 2 out]
            n238 = property on="actStatus8" class="Clust (strict)"() -> ("Value"=w258:T1)  [unwired: 2 in, 2 out]
            n239 = property on="actStatus1" class="Clust (strict)"() -> ("Value"=w251:T1)  [unwired: 2 in, 2 out]
            n240 = property on="actStatus9" class="Clust (strict)"() -> ("Value"=w259:T1)  [unwired: 2 in, 2 out]
            n241 = property on="actStatus2" class="Clust (strict)"() -> ("Value"=w252:T1)  [unwired: 2 in, 2 out]
            n242 = property on="actStatus10" class="Clust (strict)"() -> ("Value"=w260:T1)  [unwired: 2 in, 2 out]
            n243 = property on="actStatus3" class="Clust (strict)"() -> ("Value"=w253:T1)  [unwired: 2 in, 2 out]
            n244 = property on="actStatus11" class="Clust (strict)"() -> ("Value"=w261:T1)  [unwired: 2 in, 2 out]
            n245 = property on="actStatus4" class="Clust (strict)"() -> ("Value"=w254:T1)  [unwired: 2 in, 2 out]
            n246 = property on="actStatus12" class="Clust (strict)"() -> ("Value"=w262:T1)  [unwired: 2 in, 2 out]
            n247 = property on="actStatus5" class="Clust (strict)"() -> ("Value"=w255:T1)  [unwired: 2 in, 2 out]
            n248 = property on="actStatus13" class="Clust (strict)"() -> ("Value"=w263:T1)  [unwired: 2 in, 2 out]
            n249 = property on="actStatus6" class="Clust (strict)"() -> ("Value"=w256:T1)  [unwired: 2 in, 2 out]
            n250 = property on="actStatus14" class="Clust (strict)"() -> ("Value"=w264:T1)  [unwired: 2 in, 2 out]
            n251 = property on="actStatus7" class="Clust (strict)"() -> ("Value"=w257:T1)  [unwired: 2 in, 2 out]
            n252 = property on="actStatus15" class="Clust (strict)"() -> ("Value"=w265:T1)  [unwired: 2 in, 2 out]
            n253 = Unbundle By Name(w250) -> ("data"=w266:dbl[])
            n254 = Unbundle By Name(w258) -> ("data"=w281:dbl[])
            n255 = Unbundle By Name(w251) -> ("data"=w267:dbl[])
            n256 = Unbundle By Name(w259) -> ("data"=w280:dbl[])
            n257 = Unbundle By Name(w252) -> ("data"=w268:dbl[])
            n258 = Unbundle By Name(w260) -> ("data"=w279:dbl[])
            n259 = Unbundle By Name(w253) -> ("data"=w269:dbl[])
            n260 = Unbundle By Name(w261) -> ("data"=w278:dbl[])
            n261 = Unbundle By Name(w254) -> ("data"=w270:dbl[])
            n262 = Unbundle By Name(w262) -> ("data"=w277:dbl[])
            n263 = Unbundle By Name(w255) -> ("data"=w271:dbl[])
            n264 = Unbundle By Name(w263) -> ("data"=w276:dbl[])
            n265 = Unbundle By Name(w256) -> ("data"=w272:dbl[])
            n266 = Unbundle By Name(w264) -> ("data"=w275:dbl[])
            n267 = Unbundle By Name(w257) -> ("data"=w273:dbl[])
            n268 = Unbundle By Name(w265) -> ("data"=w274:dbl[])
            n269 = property on="tab" class="TabCtl (strict)"() -> ("Value"=w351:enum32{"standard"})  [unwired: 2 in, 2 out]
            n270 = call "CoreLib.stringToStringArray.vi"("String"=w355) -> ("Array"=w354:string[])
            n271 = Build Array(w266, w267, w268, w269, w270, w271, w272, w273, w281, w280, w279, w278, w277, w276, w275, w274) -> (w249:dbl[][])
            n272 = case shown="\"standard\"" w351 {
              tunnel: w354 -> [w364 _]
              tunnel: w352 -> [w363 _]
              tunnel: w318 -> [w361 _]
              tunnel: w317 -> [w362 _]
              tunnel: w315 -> [w360 _]
              tunnel: w316 -> [w359 _]
              tunnel: w282 -> [w358 _]
              tunnel: w249 -> [w357 _]
              frame "standard" {
                n273 = control-ref of="standardDisplay"() -> (w365:refnum<vi>)
                n274 = call "CSConnectGUI.update listbox.vi"("listbox"=w365, "channelNames"=w364, "nomVoltage"=w363, "actOutVoltages"=w361, "nomOutVoltages"=w358, "NumberOutChannels"=w362, "DIMInterface <> Variable"=w360, "actStatus"=w357, "ConnectionMatrix"=w359) -> ()  [unwired: 10 in, 1 out]
              }
              frame Default {
              }
            }
          }
          event Panel Close? {
            w366 = TRUE ("Discard?")
            n275 = event-data() -> ()  [unwired: 1 in, 4 out]
            n276 = event-data ("Event Filter Node")("Discard?"=w366) -> ()  [unwired: 1 in, 1 out]
          }
          event Menu Selection (User) {
            n277 = event-data() -> ("ItemTag"=w367:string)  [unwired: 1 in]
            n278 = case "menu item" shown="\"helpAboutMe\"" w367 {
              frame Default {
              }
              frame "helpAboutMe" {
                n279 = call "UtilityLib.show help.vi"("helpType"=UtilityLib.helpType."about") -> ()
              }
            }
          }
          event "Set", "plus", "minus": Value Change {
            n280 = event-data() -> ("CtlRef"=w374:refnum<vi>)  [unwired: 1 in, 5 out]
            n281 = control-ref of="Set"() -> (w378:refnum<vi>)
            n282 = control-ref of="plus"() -> (w377:refnum<vi>)
            n283 = control-ref of="minus"() -> (w376:refnum<vi>)
            n284 = Build Array(w378, w377, w376) -> (w375:refnum<vi>[])
            n285 = Search 1D Array(1D array=w375, element=w374) -> (index of element=w373:i32)  [unwired: 1 in]
            n286 = case shown="0, Default" w373 {
              tunnel: [w381 w383 w386] -> w372
              tunnel: "setValue" -> [w381 w384 w387]
              tunnel: "inc" -> [_ w382 w385]
              frame 0, Default {
                # "set"
              }
              frame 1 {
                # "plus"
                n287 = Add(x=w384, y=w382) -> (x+y=w383:dbl)
              }
              frame 2 {
                # "minus"
                n288 = Subtract(x=w387, y=w385) -> (x-y=w386:dbl)
              }
            }
            n289 = flat-sequence {
              tunnel: w372 -> [w379]
              tunnel: w369 -> [w380]
              frame #0 {
                n290 = property on="setValue" class="DigNum (strict)"("Value"=w379) -> ()  [unwired: 2 in, 2 out]
              }
              frame #1 {
                n291 = Set Occurrence(w380) -> ()
              }
            }
          }
          event "EmergencyOff": Value Change {
            n292 = event-data() -> ()  [unwired: 1 in, 6 out]
            n293 = call "CSConnectGUI.EmergencyOff.vi"("i ref in"=w388) -> ()  [unwired: 17 in, 2 out]
          }
          event Value Change {
            n294 = event-data() -> ()  [unwired: 1 in, 6 out]
            n295 = Unbundle By Name("deviceID") -> ("data"=w391:string)
            n296 = call "UtilityLib.remove white spaces.vi"("string with blanks"=w391) -> ("string without white spaces"=→"deviceIDString":string)  [unwired: 14 in, 4 out]
          }
          event Value Change {
            n297 = event-data() -> ()  [unwired: 1 in, 6 out]
            n298 = Unbundle By Name("state") -> ("no link"=w395:bool, "data"=w394:dbl)
            n299 = call "DeviceBase.device state 2 value status.vi"("deviceState"=w394, "no link"=w395) -> ("valueStatus"=w393:T4)
            n300 = call "UtilityLib.Sixcolor.vi"("State"=w393) -> ("elementBackground"=w397:u32, "elementText"=w392:u32)  [unwired: 2 in, 2 out]
            n301 = property on="deviceIDString" class="Str"("Text.BGColor"=w397, "Text.TextColor"=w392) -> ()  [unwired: 2 in, 2 out]
          }
          event Value Change {
            n302 = event-data() -> ()  [unwired: 1 in, 6 out]
            n303 = Unbundle By Name("nofChannels") -> ("no link"=w400:bool, "data"=w406:dbl)
            n304 = To Long Integer(number=w406) -> (32bit integer=w401:i32)
            n305 = Select(t=0, s=w400, f=w401) -> (s? t:f=w399:i32)
            n306 = property on="standardDisplay" class="MCListbox (strict)"() -> (error out=w407:errorcluster, "ItemNames"=w413:string[][])  [unwired: 2 in, 1 out]
            n307 = for "pre-coloring for channels" {
              N: w399 -> [_]
              tunnel: [w420] -> w404
              i -> [w419]
              n308 = Bundle(w419, -2) -> (w421:cluster{i32, i32})  [unwired: 1 in]
              n309 = call "UtilityLib.Sixcolor.vi"("State"=UtilityLib.valueStatus."control default" ("valueStatus")) -> ("elementBackground"=w418:u32, "elementText"=w417:u32)  [unwired: 2 in, 2 out]
              n310 = property on="standardDisplay" class="MCListbox (strict)"("ActiveCell"=w421, "CellBG"=w418, "CellFontColor"=w417) -> (error out=w420:errorcluster)  [unwired: 2 in, 1 out]
            }
            n311 = Array Size(array=w413) -> (size(s)=w411:i32[])
            n312 = Index Array(array=w411) -> (element #1=w410:i32, element #2=w409:i32)  [unwired: 2 in]
            n313 = flat-sequence {
              frame #0 {
                n314 = Wait (ms)(milliseconds to wait=u32 500) -> ()  [unwired: 1 out]
              }
              frame #1 {
                n315 = property on="function" class="Ring (strict)"() -> ("Value"=w415:u16)  [unwired: 2 in, 2 out]
                n316 = property on="function" class="Ring (strict)"("Val(Sgnl)"=w415) -> ()  [unwired: 2 in, 2 out]
              }
            }
            n317 = Initialize Array("" ("Empty String Constant"), w410, w409) -> (w408:string[][])
            n318 = property on="standardDisplay" class="MCListbox (strict)"(error in=w407, "ItemNames"=w408) -> ()  [unwired: 1 in, 2 out]
            n319 = for "coloring of an arbitrary number of following lines" {
              N: 16 -> [_]
              tunnel: w399 -> [w431]
              tunnel: w404 -> [w426]
              i -> [w430]
              n320 = Add(x=w431, y=w430) -> (x+y=w429:i32)
              n321 = Bundle(w429, -2) -> (w427:cluster{i32, i32})  [unwired: 1 in]
              n322 = call "UtilityLib.Sixcolor.vi"("State"=UtilityLib.valueStatus."system default" ("valueStatus")) -> ("elementBackground"=w424:u32, "elementText"=w423:u32)  [unwired: 2 in, 2 out]
              n323 = property on="standardDisplay" class="MCListbox (strict)"(error in=w426, "ActiveCell"=w427, "CellBG"=w424, "CellFontColor"=w423) -> ()  [unwired: 1 in, 2 out]
            }
            n324 = property on="channelIndex" class="DigNum (strict)"("Value"=u16 0 ("channelIndex")) -> ()  [unwired: 2 in, 2 out]
          }
          event "standardDisplay": Value Change {
            n325 = event-data() -> ("NewVal"=w432:i32[])  [unwired: 1 in, 5 out]
            n326 = Array Size(array=w432) -> (size(s)=w433:i32)
            n327 = case shown="1, Default" w433 {
              tunnel: w432 -> [_ w439]
              frame 0 {
              }
              frame 1, Default {
                # "trigger function event\nto update the set value"
                n328 = Index Array(array=w439, index=0) -> (element=w434:i32)
                n329 = property on="channelIndex" class="DigNum (strict)"("Value"=w434) -> (error out=w435:errorcluster)  [unwired: 2 in, 1 out]
                n330 = property on="function" class="Ring (strict)"(error in=w435) -> (error out=w436:errorcluster, "Value"=w437:u16)  [unwired: 1 in, 1 out]
                n331 = property on="function" class="Ring (strict)"(error in=w436, "Val(Sgnl)"=w437) -> ()  [unwired: 1 in, 2 out]
              }
            }
          }
          event "function": Value Change {
            n332 = event-data() -> ()  [unwired: 1 in, 6 out]
            n333 = property on="function" class="Ring (strict)"() -> ("Strings []"=w446:string[])  [unwired: 2 in, 2 out]
            n334 = To Long Integer(number="function") -> (32bit integer=w447:i32)
            n335 = property on="standardDisplay" class="MCListbox (strict)"() -> ("Value"=w450:i32[])  [unwired: 2 in, 2 out]
            n336 = Index Array(array=w446, index=w447) -> (element=w444:string)
            n337 = Index Array(array=w450, index=0) -> (element=w448:i32)
            n338 = Search 1D Array(1D array=w443, element=w444) -> (index of element=w442:i32)  [unwired: 1 in]
            n339 = case shown="0, Default" w442 {
              tunnel: w448 -> [w455 _]
              tunnel: "function" -> [w454 _]
              tunnel: w441 -> [w452 _]
              tunnel: w440 -> [w451 _]
              frame 0, Default {
                w453 = u8 0 ("Disabled")
                n340 = case shown="1" w454 {
                  tunnel: [w458 w459 w515] -> w457
                  tunnel: [w458 1.0 w516] -> w456
                  tunnel: w455 -> [_ w466 w518]
                  tunnel: w452 -> [_ w467 _]
                  tunnel: w451 -> [_ w464 _]
                  frame 0, Default {
                    w458 = inf ("Positive Infinity")
                  }
                  frame 1 {
                    n341 = property on="actStatus0" class="Clust (strict)"() -> ("Value"=w499:T1)  [unwired: 2 in, 2 out]
                    n342 = property on="actStatus8" class="Clust (strict)"() -> ("Value"=w491:T1)  [unwired: 2 in, 2 out]
                    n343 = property on="actStatus1" class="Clust (strict)"() -> ("Value"=w498:T1)  [unwired: 2 in, 2 out]
                    n344 = property on="actStatus9" class="Clust (strict)"() -> ("Value"=w490:T1)  [unwired: 2 in, 2 out]
                    n345 = property on="actStatus10" class="Clust (strict)"() -> ("Value"=w489:T1)  [unwired: 2 in, 2 out]
                    n346 = property on="actStatus2" class="Clust (strict)"() -> ("Value"=w497:T1)  [unwired: 2 in, 2 out]
                    n347 = property on="actStatus3" class="Clust (strict)"() -> ("Value"=w496:T1)  [unwired: 2 in, 2 out]
                    n348 = property on="actStatus11" class="Clust (strict)"() -> ("Value"=w488:T1)  [unwired: 2 in, 2 out]
                    n349 = property on="actStatus12" class="Clust (strict)"() -> ("Value"=w487:T1)  [unwired: 2 in, 2 out]
                    n350 = property on="actStatus4" class="Clust (strict)"() -> ("Value"=w495:T1)  [unwired: 2 in, 2 out]
                    n351 = property on="actStatus5" class="Clust (strict)"() -> ("Value"=w494:T1)  [unwired: 2 in, 2 out]
                    n352 = property on="actStatus13" class="Clust (strict)"() -> ("Value"=w486:T1)  [unwired: 2 in, 2 out]
                    n353 = property on="actStatus6" class="Clust (strict)"() -> ("Value"=w493:T1)  [unwired: 2 in, 2 out]
                    n354 = property on="actStatus14" class="Clust (strict)"() -> ("Value"=w485:T1)  [unwired: 2 in, 2 out]
                    n355 = property on="actStatus7" class="Clust (strict)"() -> ("Value"=w492:T1)  [unwired: 2 in, 2 out]
                    n356 = property on="actStatus15" class="Clust (strict)"() -> ("Value"=w484:T1)  [unwired: 2 in, 2 out]
                    n357 = Index Array(array=w467, index (row)=w466) -> (element=w465:bool[])  [unwired: 1 in]
                    n358 = Unbundle By Name(w491) -> ("data"=w468:dbl[])
                    n359 = Unbundle By Name(w499) -> ("data"=w483:dbl[])
                    n360 = Unbundle By Name(w490) -> ("data"=w469:dbl[])
                    n361 = Unbundle By Name(w498) -> ("data"=w482:dbl[])
                    n362 = Unbundle By Name(w489) -> ("data"=w470:dbl[])
                    n363 = Unbundle By Name(w497) -> ("data"=w481:dbl[])
                    n364 = Unbundle By Name(w488) -> ("data"=w471:dbl[])
                    n365 = Unbundle By Name(w496) -> ("data"=w480:dbl[])
                    n366 = Unbundle By Name(w487) -> ("data"=w472:dbl[])
                    n367 = Unbundle By Name(w495) -> ("data"=w479:dbl[])
                    n368 = Unbundle By Name(w486) -> ("data"=w473:dbl[])
                    n369 = Unbundle By Name(w494) -> ("data"=w478:dbl[])
                    n370 = Unbundle By Name(w485) -> ("data"=w474:dbl[])
                    n371 = Unbundle By Name(w493) -> ("data"=w477:dbl[])
                    n372 = Unbundle By Name(w484) -> ("data"=w475:dbl[])
                    n373 = Unbundle By Name(w492) -> ("data"=w476:dbl[])
                    n374 = Build Array(w483, w482, w481, w480, w479, w478, w477, w476, w468, w469, w470, w471, w472, w473, w474, w475) -> (w463:dbl[][])
                    n375 = for {
                      tunnel: w465 -> [w504] mode=indexing
                      tunnel: w464 -> [w503] mode=indexing
                      tunnel: w463 -> [w502]
                      tunnel: [w501] -> w462 mode=indexing
                      n376 = case shown="True" w504 {
                        tunnel: w503 -> [_ w513]
                        tunnel: w502 -> [_ w514]
                        tunnel: [TRUE w506] -> w501
                        frame False {
                        }
                        frame True {
                          n377 = Unbundle By Name(w513) -> ("ObjectIndex"=w511:i32, "OutChannelIndex"=w512:i32)
                          n378 = Index Array(array=w514, index (row)=w511, index (col)=w512) -> (element=w510:dbl)
                          n379 = To Long Integer(number=w510) -> (32bit integer=w509:i32)
                          n380 = Number To Boolean Array(number=w509) -> (Boolean array=w508:bool[])
                          n381 = Index Array(array=w508, index=0) -> (element=w506:bool)
                        }
                      }
                    }
                    n382 = And Array Elements(Boolean array=w462) -> (logical AND=w460:bool)
                    n383 = Boolean To (0,1)(Boolean=w460) -> (0, 1=w461:i16)
                    n384 = To Double Precision Float(number=w461) -> (double precision float=w459:dbl)
                  }
                  frame 2 {
                    n385 = property on="nomVoltage" class="Clust (strict)"() -> ("Value"=w519:T1)  [unwired: 2 in, 2 out]
                    n386 = Unbundle By Name(w519) -> ("data"=w517:dbl[])
                    n387 = Index Array(array=w517, index=w518) -> (element=w515:dbl)
                    n388 = call "UtilityLib.guess increment from number.vi"("number"=w515) -> ("increment"=w516:dbl)
                  }
                }
                n389 = property on="setValue" class="DigNum (strict)"("Value"=w457) -> ()  [unwired: 2 in, 2 out]
                n390 = property on="inc" class="DigNum (strict)"("Value"=w456) -> ()  [unwired: 2 in, 2 out]
                n391 = property on="Set" class="Bool"("Disabled"=w453) -> ()  [unwired: 2 in, 2 out]
                n392 = property on="plus" class="Bool"("Disabled"=w453) -> ()  [unwired: 2 in, 2 out]
                n393 = property on="minus" class="Bool"("Disabled"=w453) -> ()  [unwired: 2 in, 2 out]
              }
              frame -1 {
                w520 = u8 2 ("Disabled")
                n394 = property on="Set" class="Bool"("Disabled"=w520) -> ()  [unwired: 2 in, 2 out]
                n395 = property on="plus" class="Bool"("Disabled"=w520) -> ()  [unwired: 2 in, 2 out]
                n396 = property on="minus" class="Bool"("Disabled"=w520) -> ()  [unwired: 2 in, 2 out]
              }
            }
          }
        }
        "loop counter" <- w247
      }
    }
    frame #6 {
      n397 = property on="Property Node" class="VI"() -> ("Front Panel.PanelBounds"=w524:T12)  [unwired: 2 in, 2 out]
      n398 = Unbundle By Name(w524) -> ("Left"=w522:i16)
      n399 = Add(x=w522, y=i16 287) -> (x+y=w521:i16)
      n400 = for {
        tunnel: w526 -> [w527] mode=indexing
        n401 = call "DimIndicators.dic_release_service.vi"("controlRef"=w527) -> ()  [unwired: 18 in, 1 out]
      }
      n402 = Bundle By Name(cluster=w524, "Right"=w521) -> (w523:T12)
      n403 = property on="Property Node" class="VI"("Front Panel.PanelBounds"=w523) -> ()  [unwired: 2 in, 2 out]
    }
    frame #7 {
      n404 = call "DeviceBaseGUI.close panel.vi"("i ref in"=w528) -> ()  [unwired: 17 in, 2 out]
    }
  }
  n405 = while {
    tunnel: w53 -> [w533]
    tunnel: "object ref" -> [w531]
    stop <- FALSE stop-if-true
    n406 = Wait on Occurrence(1:FALSE ("ignore previous (T)"), 2:w533) -> (0:w532:bool)  [unwired: 1 in]
    n407 = flat-sequence {
      tunnel: w532 -> [_]
      tunnel: w531 -> [w536]
      tunnel: [w536] -> w530
      tunnel: w530 -> [w541]
      tunnel: [w540] -> w529
      tunnel: w529 -> [w554]
      frame #0 {
        n408 = property on="Busy" class="Bool (strict)"("Blinking"=TRUE) -> ()  [unwired: 2 in, 2 out]
      }
      frame #1 {
        n409 = property on="function" class="Ring (strict)"() -> ("Value"=w548:u16)  [unwired: 2 in, 2 out]
        n410 = property on="function" class="Ring (strict)"() -> ("Strings []"=w547:string[])  [unwired: 2 in, 2 out]
        n411 = property on="setValue" class="DigNum (strict)"() -> ("Value"=w545:dbl)  [unwired: 2 in, 2 out]
        n412 = Index Array(array=w547, index=w548) -> (element=w542:string)
        n413 = property on="standardDisplay" class="MCListbox (strict)"() -> ("Value"=w538:i32[])  [unwired: 2 in, 2 out]
        n414 = case shown="1" w548 {
          tunnel: [w550 w553] -> w539
          tunnel: w545 -> [w549 w552]
          frame 0, Default {
            n415 = call-poly "CoreLib.data 2 byte array.vi"("f64"=w549) -> ("byteArray out"=w550:T13)  [unwired: 18 in]
          }
          frame 1 {
            n416 = To Word Integer(number=w552) -> (16bit integer=w551:i16)
            n417 = call-poly "CoreLib.data 2 byte array.vi"("i16"=w551) -> ("byteArray out"=w553:T13)  [unwired: 18 in]
          }
        }
        n418 = call "DeviceBaseGUI.set channel value.vi"("i ref in"=w541, "byteArray"=w539, "methodName"=w542, "channels"=w538) -> ("error out"=w544:errorcluster)  [unwired: 14 in, 1 out]
        n419 = Unbundle By Name(w544) -> ("code"=w546:i32, "status"=w540:bool)
        n420 = call "CoreLib.get error string.vi"("Error Code"=w546) -> ("Error String"=w543:string)
        n421 = local write "ErrorString"(w543) -> ()
      }
      frame #2 {
        n422 = property on="Busy" class="Bool (strict)"("Value"=w554, "Blinking"=FALSE) -> ()  [unwired: 2 in, 2 out]
      }
    }
  }
